vi "HGF_Composite.appendData2Variant.vi"(0 "initData":variant, 2 "Components":refnum<class "HGF_Component.lvclass">[](array[class]), 5 "error in (no error)":errorcluster) -> (14 "dup initData":variant, 19 "error out":errorcluster)   [LabVIEW 2014, in "HGF_BaseClasses.lvlib" / "HGF_Composite.lvclass"]
uses:
  HGF_Composite.lvclass
  HGF_Component/HGF_Component.lvclass
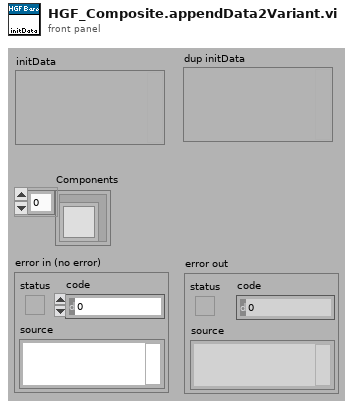
[diagram p1: front panel]
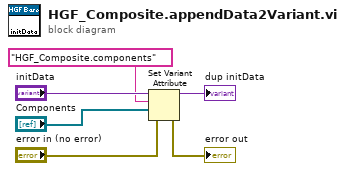
[diagram p0: block diagram]
diagram:
  n1 = Set Variant Attribute(Variant="initData", name="HGF_Composite.components", value="Components", error in="error in (no error)") -> (Variant out=→"dup initData":variant, error out=→"error out":errorcluster)  [unwired: 1 out]
